vi "Get Instrument Info Array from Connection Map.vi"(10 "Pin Names for Scope":string[](array[string]), 11 "connection map":map{string, T1[]}(c390)) -> (3 "instrument info array":T1[](array[typedef]))   [LabVIEW 2021, in "PMIC Common.lvlib"]
uses:
  PMIC Common.lvlib
  Instrument Info.ctl
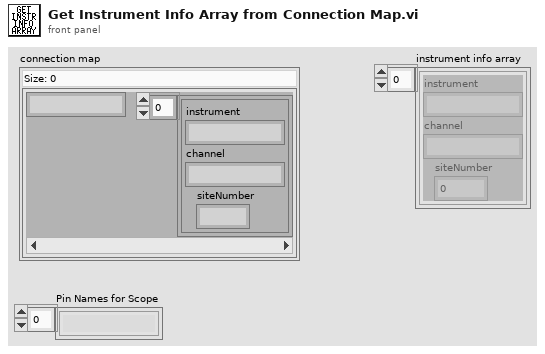
[diagram p1: front panel]
types:
  T1 = typedef "PMIC Common.lvlib/Instrument Info.ctl" = cluster{"instrument":string, "channel":string, "siteNumber":i32}
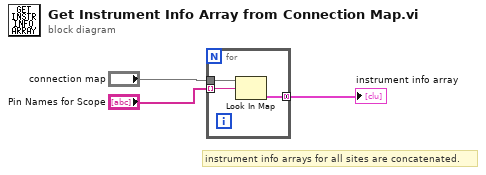
[diagram p0: block diagram]
diagram:
  # "instrument info arrays for all sites are concatenated."
  n1 = for {
    tunnel: "connection map" -> [w6]
    tunnel: "Pin Names for Scope" -> [w5] mode=indexing
    tunnel: [w4] -> w1 mode=concatenating
    n2 = Look In Map(map=w6, key=w5) -> (value=w4:T1[])  [unwired: 1 in, 1 out]
  }
  "instrument info array" <- w1
